vi "File-Generator Module.vi"(11 "Metadata for all trials/volumes":T1[](array[typedef])=[{"Imaging Protocol"=enum."Functional Acquisition", "Number of Trials"=2, "Frame Size"=512, "# Averaged frames"=1, "Dwell time (us)"=0.1, "Index of Z-plane"=0, "Timelapse?"=FALSE, "Logging process is active"=TRUE, "Speed logging enabled"=FALSE, "tdms file ref"=refnum, "path"=path "E:/UCL/Rig 3 MovCor integration version/Datasets/Dual Plane datasets/150701_01_13_28/Functional imaging TDMS data files/001.tdms", "Trial Number"=1, "Expected # points acquired"=TRUE, "Manually stopped"=FALSE, "Last trial"=FALSE, "Ch0 data"=[], "Ch1 data"=[], "Ref Data"=[], "Ref Frame Time"=[], "Image Time"=[], "Continuous Time"=[], "Ref X Length"=0, "Ref Y Length"=0, "# Ref Averaged frames"=1, "Ref Dwell time (us)"=0.20000000298023224, "Points acquired"={"Ch0 last trial"=34078720, "Ch1 last trial"=34078720, "All trials"=34078720}, "HW Timings File"=refnum}, {"Imaging Protocol"=enum."Functional Acquisition", "Number of Trials"=2, "Frame Size"=512, "# Averaged frames"=1, "Dwell time (us)"=0.1, "Index of Z-plane"=0, "Timelapse?"=FALSE, "Logging process is active"=TRUE, "Speed logging enabled"=FALSE, "tdms file ref"=refnum, "path"=path "E:/UCL/Rig 3 MovCor integration version/Datasets/Dual Plane datasets/150701_01_13_28/Functional imaging TDMS data files/002.tdms", "Trial Number"=2, "Expected # points acquired"=TRUE, "Manually stopped"=FALSE, "Last trial"=TRUE, "Ch0 data"=[], "Ch1 data"=[], "Ref Data"=[], "Ref Frame Time"=[], "Image Time"=[], "Continuous Time"=[], "Ref X Length"=0, "Ref Y Length"=0, "# Ref Averaged frames"=1, "Ref Dwell time (us)"=0.20000000298023224, "Points acquired"={"Ch0 last trial"=34078720, "Ch1 last trial"=34078720, "All trials"=68157440}, "HW Timings File"=refnum}, {"Imaging Protocol"=enum."Functional Acquisition", "Number of Trials"=2, "Frame Size"=512, "# Averaged frames"=1, "Dwell time (us)"=0.1, "Index of Z-plane"=0, "Timelapse?"=FALSE, "Logging process is active"=TRUE, "Speed logging enabled"=FALSE, "tdms file ref"=refnum, "path"=path "E:/UCL/Rig 3 MovCor integration version/Datasets/Dual Plane datasets/150701_01_13_28/Functional imaging TDMS data files/003.tdms", "Trial Number"=2, "Expected # points acquired"=TRUE, "Manually stopped"=FALSE, "Last trial"=TRUE, "Ch0 data"=[], "Ch1 data"=[], "Ref Data"=[], "Ref Frame Time"=[], "Image Time"=[], "Continuous Time"=[], "Ref X Length"=0, "Ref Y Length"=0, "# Ref Averaged frames"=1, "Ref Dwell time (us)"=0.20000000298023224, "Points acquired"={"Ch0 last trial"=34078720, "Ch1 last trial"=34078720, "All trials"=68157440}, "HW Timings File"=refnum}] {"Ref Dwell time (us)" format="%#.6g"; "Frame Size" items=["100X100"=100, "128X128"=128, "200X200"=200, "256X256"=256, "512X512"=512, "1024x1024"=1024, "2048x2048"=2048]; "Dwell time (us)" format="%#.6g"}) -> ()   [LabVIEW 2020]
uses:
  Typedefs/Logging queue element.ctl
  Typedefs/Imaging Protocols enum.ctl
  Typedefs/Frame Size.ctl
  Typedefs/Acquired points count.ctl
  Typedefs/Top level VI states.ctl
  Global Variables/General Globals.vi
  Global Variables/gl_Queues.vi
panel:
  out "Continuous Time":u64[][](array[numeric])
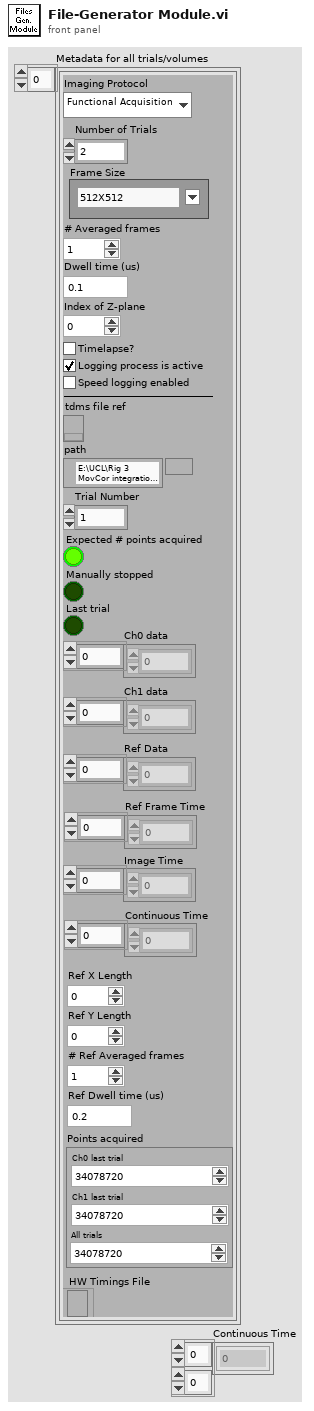
[diagram p1: front panel]
types:
  T1 = typedef "Logging queue element.ctl" = cluster{"Imaging Protocol":T2, "Number of Trials":u16, "Frame Size":T3, "# Averaged frames":u16, "Dwell time (us)":dbl, "Index of Z-plane":i32, "Timelapse?":bool, "Logging process is active":bool, "Speed logging enabled":bool, "tdms file ref":refnum<k34>, "path":path, "Trial Number":i32, "Expected # points acquired":bool, "Manually stopped":bool, "Last trial":bool, "Ch0 data":u32[], "Ch1 data":u32[], "Ref Data":u32[], "Ref Frame Time":u64[], "Image Time":u64[], "Continuous Time":u64[], "Ref X Length":u16, "Ref Y Length":u16, "# Ref Averaged frames":u16, "Ref Dwell time (us)":dbl, "Points acquired":T4, "HW Timings File":refnum<file>}
  T2 = typedef "Imaging Protocols enum.ctl" = enum16{"AOL Z-Stack", "Motor Z Stack", "Functional Acquisition", "Single Plane Acquisition", "Volume Acquisition", "Live Imaging", "Live Plane Imaging", "Live Volume Imaging"}
  T3 = typedef "Frame Size.ctl" = u16
  T4 = typedef "Acquired points count.ctl" = cluster{"Ch0 last trial":u64, "Ch1 last trial":u64, "All trials":u64}
  T5 = typedef "Top level VI states.ctl" = enum16{"None", "Initialise UI", "<STACK PROTOCOL STATES>", "AOL Zstack-START", "AOL Zstack-STOP", "Motor Zstack-START", "Motor Zstack-STOP", "<ACQUISITION PROTOCOL STATES> ", "Functional Acquisition-START", "Functional Acquisition-STOP", "Single Plane Acquisition-START", "Single Plane Acquisition-STOP", "Volume Acquisition-START", "Volume Acquisition-STOP", "<LIVE IMAGING PROTOCOL STATES>", "Live Imaging-START", "Live Imaging-STOP", "Live Plane Imaging-START", "Live Plane Imaging-STOP", "Live Volume Imaging-START", "Live Volume Imaging-STOP", "<MOVEMENT CORRECTION PROTOCOL STATES>", "EXIT"}
  T6 = typedef "All Message Queues.ctl" = cluster{"UI queue":refnum<queue>, "Acq. queue":refnum<queue>, "Logging queue":refnum<queue>}
  T7 = typedef "ROI ID Enum.ctl" = enum16{"Point", "MiniScan", "Comp. MiniScan", "Rectangle", "Comp. volume", "Arb. plane point", "None"}
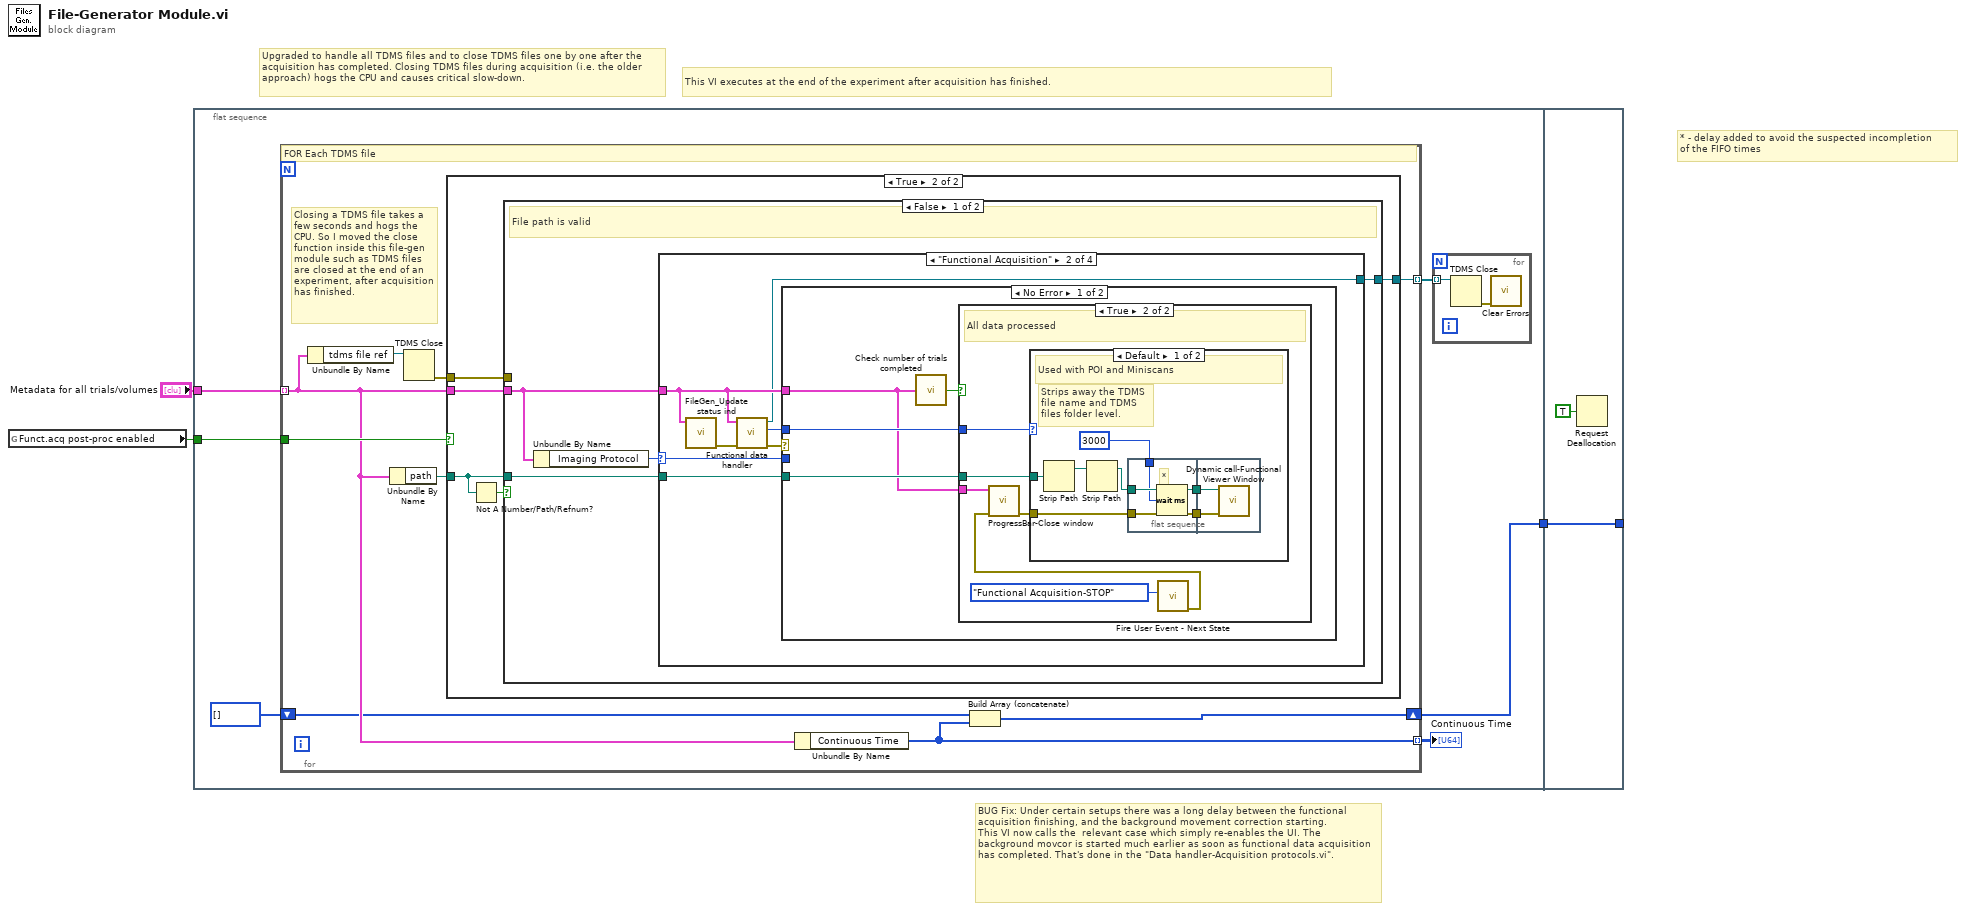
[diagram p0: block diagram]
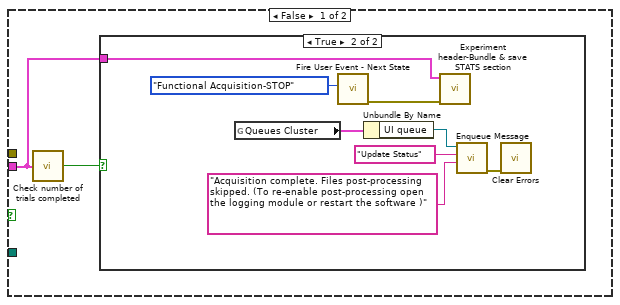
[diagram p2: hidden frame]
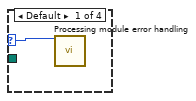
[diagram p4: hidden frame]
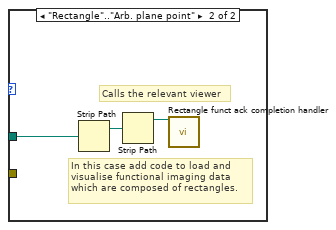
[diagram p6: hidden frame]
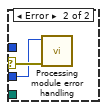
[diagram p7: hidden frame]
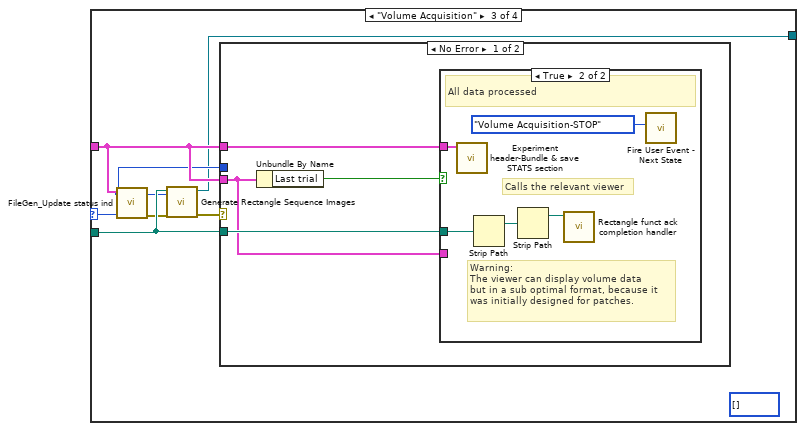
[diagram p8: hidden frame]
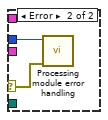
[diagram p10: hidden frame]
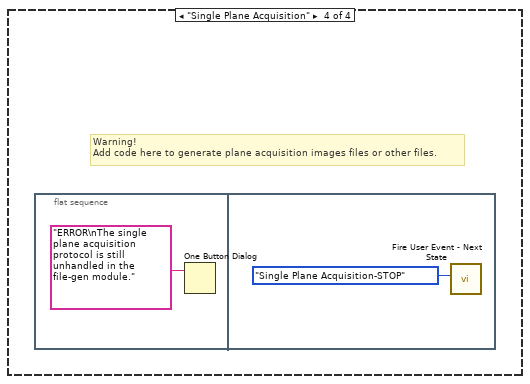
[diagram p11: hidden frame]
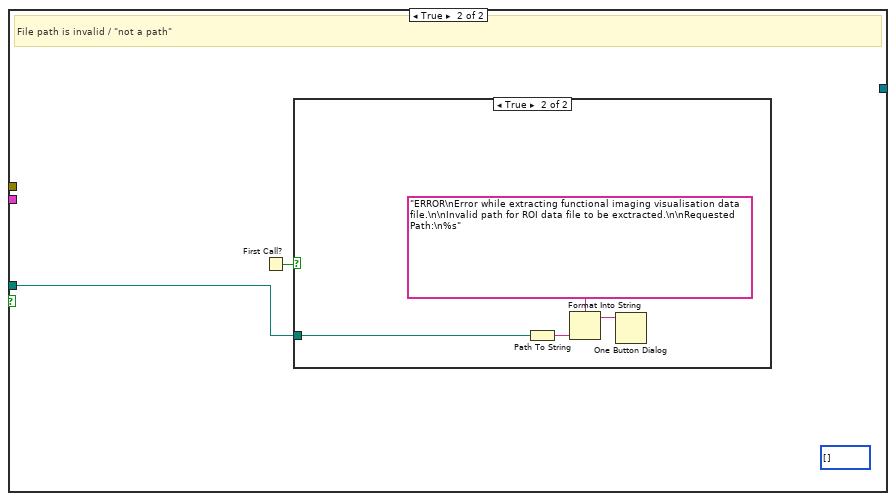
[diagram p12: hidden frame]
diagram:
  # "* - delay added to avoid the suspected incompletion\nof the FIFO times"
  # "BUG Fix: Under certain setups there was a long delay between the functional acquisition finishing, and the background movement correction starting.\nThis VI now calls the  relevant case which simply re-enables the UI. The background movcor is started much earlier as soon as functional data acquisition has completed. That's done in the \"Data handler-Acquisition protocols.vi\"."
  # "This VI executes at the end of the experiment after acquisition has finished."
  # "Upgraded to handle all TDMS files and to close TDMS files one by one after the acquisition has completed. Closing TDMS files during acquisition (i.e. the older approach) hogs the CPU and causes critical slow-down."
  n1 = global read "General Globals.vi" "Funct.acq post-proc enabled"() -> (w2:bool)
  n2 = flat-sequence {
    tunnel: "Metadata for all trials/volumes" -> [w9]
    tunnel: w2 -> [w8]
    tunnel: [w5] -> w1
    tunnel: [w100] -> _
    tunnel: w1 -> [w100]
    frame #0 {
      n3 = for {
        tunnel: w9 -> [w15] mode=indexing
        tunnel: w8 -> [w17]
        tunnel: [w16] -> w7 mode=indexing
        shift-right: [w13] -> w5
        shift-left: u64[] [] -> [w14]
        tunnel: [w12] -> w4 mode=indexing
        # "Closing a TDMS file takes a few seconds and hogs the CPU. So I moved the close function inside this file-gen module such as TDMS files are closed at the end of an experiment, after acquisition has finished."
        # "FOR Each TDMS file"
        n4 = Unbundle By Name(w15) -> ("tdms file ref"=w19:refnum<k34>)
        n5 = Unbundle By Name(w15) -> ("path"=w20:path)
        n6 = TDMS Close(11:w19) -> (0:w18:errorcluster)  [unwired: 1 in, 1 out]
        n7 = case shown="True" w17 {
          tunnel: w20 -> [_ w35]
          tunnel: w15 -> [w21 w34]
          tunnel: w18 -> [_ w33]
          tunnel: [_ w31] -> w16
          frame False {
            n8 = call "Check number of trials completed.vi"("Cluster"=w21) -> ("# of trials completed"=w22:bool)
            n9 = case shown="True" w22 {
              tunnel: w21 -> [_ w23]
              frame False {
              }
              frame True {
                n10 = global read "gl_Queues.vi" "Queues Cluster"() -> (w28:T6)
                n11 = call "Fire User Event - Next State.vi"("\"UI Handler loop\" case to execute"=Top_level_VI_states."Functional Acquisition-STOP" ("event data / imaging mode")) -> ("Error Out"=w24:errorcluster)  [unwired: 10 in]
                n12 = Unbundle By Name(w28) -> ("UI queue"=w27:refnum<queue>)
                n13 = call "Experiment header-Bundle & save STATS section.vi"("error in (no error)"=w24, "Logging queue element"=w23) -> ()  [unwired: 9 in, 1 out]
                n14 = call "Enqueue Message.vi"("Message Data"="Acquisition complete. Files post-processing skipped. (To re-enable post-processing open the logging module or restart the software )" ("Acquiring and Logging..."), "Message"="Update Status", "Queue"=w27) -> ("error out"=w26:errorcluster)  [unwired: 7 in, 1 out]
                n15 = call <vilib>:"Clear Errors.vi"("error in (no error)"=w26) -> ()  [unwired: 5 in, 2 out]
              }
            }
          }
          frame True {
            n16 = Not A Number/Path/Refnum?(number/path/refnum=w35) -> (NaN/Path/Refnum?=w32:bool)
            n17 = case shown="False" w32 {
              tunnel: w35 -> [w39 w95]
              tunnel: w34 -> [w37 _]
              tunnel: w33 -> [_ _]
              tunnel: [w36 _] -> w31
              frame False {
                # "File path is valid"
                n18 = Unbundle By Name(w37) -> ("Imaging Protocol"=w38:T2)
                n19 = case shown="\"Functional Acquisition\"" w38 {
                  selector: w38 -> [w40 w42 w76 _]
                  tunnel: w37 -> [_ w43 w77 _]
                  tunnel: w39 -> [_ w46 w80 _]
                  tunnel: [_ w41 w75 _] -> w36
                  frame Default {
                    n20 = call "Processing module error handling.vi"("Imaging Protocol"=w40) -> ()  [unwired: 11 in]
                  }
                  frame "Functional Acquisition" {
                    n21 = call "FileGen_Update status ind.vi"("Cluster"=w43) -> ("error out"=w44:errorcluster)  [unwired: 10 in]
                    n22 = call "Functional data handler.vi"("error in"=w44, "Setup cluster"=w43) -> ("error out"=w47:errorcluster, "Predominant ROI type"=w45:T7, "tdms file to close"=w41:refnum<k34>)  [unwired: 6 in, 1 out]
                    n23 = case shown="No Error" w47 {
                      selector: w47 -> [_ w74]
                      tunnel: w46 -> [w50 _]
                      tunnel: w43 -> [w48 _]
                      tunnel: w45 -> [w49 _]
                      tunnel: w42 -> [_ w73]
                      frame No Error {
                        n24 = call "Check number of trials completed.vi"("Cluster"=w48) -> ("# of trials completed"=w51:bool)
                        n25 = case shown="True" w51 {
                          tunnel: w50 -> [_ w57]
                          tunnel: w48 -> [_ w55]
                          tunnel: w49 -> [_ w56]
                          frame False {
                            # "Still processing..."
                          }
                          frame True {
                            # "All data processed"
                            n26 = call "Fire User Event - Next State.vi"("\"UI Handler loop\" case to execute"=Top_level_VI_states."Functional Acquisition-STOP" ("event data / imaging mode")) -> ("Error Out"=w52:errorcluster)  [unwired: 10 in]
                            n27 = call "ProgressBar-Close window.vi"("error in"=w52, "Z-stack queue cluster"=w55) -> ("error out (no error)"=w53:errorcluster)  [unwired: 9 in]
                            n28 = case shown="Default" w56 {
                              tunnel: w57 -> [w63 w71]
                              tunnel: w53 -> [w62 _]
                              frame Default {
                                # "Strips away the TDMS file name and TDMS files folder level."
                                # "Used with POI and Miniscans"
                                n29 = Strip Path(path=w63) -> (stripped path=w64:path)  [unwired: 1 out]
                                n30 = Strip Path(path=w64) -> (stripped path=w61:path)  [unwired: 1 out]
                                n31 = flat-sequence {
                                tunnel: w61 -> [w66]
                                tunnel: w62 -> [w67]
                                tunnel: [w67] -> w60
                                tunnel: [w66] -> w59
                                tunnel: u32 3000 -> [w65]
                                tunnel: w60 -> [w69]
                                tunnel: w59 -> [w68]
                                frame #0 {
                                # "*"
                                n32 = Wait (ms)(milliseconds to wait=w65) -> ()  [unwired: 1 out]
                                }
                                frame #1 {
                                n33 = call "Dynamic call-Functional Viewer Window.vi"("error in (no error)"=w69, "Experiment data folder path"=w68) -> ()  [unwired: 10 in]
                                }
                                }
                              }
                              frame "Rectangle".."Arb. plane point" {
                                # "Calls the relevant viewer"
                                # "In this case add code to load and visualise functional imaging data which are composed of rectangles."
                                n34 = Strip Path(path=w71) -> (stripped path=w72:path)  [unwired: 1 out]
                                n35 = Strip Path(path=w72) -> (stripped path=w70:path)  [unwired: 1 out]
                                n36 = call "Rectangle funct ack completion handler.vi"("Destination folder"=w70) -> ()  [unwired: 11 in]
                              }
                            }
                          }
                        }
                      }
                      frame Error {
                        n37 = call "Processing module error handling.vi"("error in (no error)"=w74, "Imaging Protocol"=w73) -> ()  [unwired: 10 in]
                      }
                    }
                  }
                  frame "Volume Acquisition" {
                    (unwired) u64[] [] ("Continuous Time")
                    n38 = call "FileGen_Update status ind.vi"("Cluster"=w77) -> ("error out"=w78:errorcluster)  [unwired: 10 in]
                    n39 = call "Generate Rectangle Sequence Images.vi"("Imaging Protocol"=w76, "error in (no error)"=w78, "TDMS file path & name"=w80) -> ("error out"=w79:errorcluster, "tdms file to close"=w75:refnum<k34>)  [unwired: 6 in, 1 out]
                    n40 = case shown="No Error" w79 {
                      selector: w79 -> [_ w91]
                      tunnel: w80 -> [w84 _]
                      tunnel: w77 -> [w83 _]
                      tunnel: w77 -> [w81 _]
                      tunnel: w76 -> [_ w90]
                      frame No Error {
                        n41 = Unbundle By Name(w83) -> ("Last trial"=w82:bool)
                        n42 = case shown="True" w82 {
                          tunnel: w84 -> [_ w85]
                          tunnel: w83 -> [_ _]
                          tunnel: w81 -> [_ w88]
                          frame False {
                            # "Still processing..."
                          }
                          frame True {
                            # "Warning:\nThe viewer can display volume data\nbut in a sub optimal format, because it\nwas initially designed for patches."
                            # "Calls the relevant viewer"
                            # "All data processed"
                            n43 = call "Experiment header-Bundle & save STATS section.vi"("Logging queue element"=w88) -> ()  [unwired: 10 in, 1 out]
                            n44 = Strip Path(path=w85) -> (stripped path=w87:path)  [unwired: 1 out]
                            n45 = Strip Path(path=w87) -> (stripped path=w86:path)  [unwired: 1 out]
                            n46 = call "Rectangle funct ack completion handler.vi"("Destination folder"=w86) -> ()  [unwired: 11 in]
                            n47 = call "Fire User Event - Next State.vi"("\"UI Handler loop\" case to execute"=Top_level_VI_states."Volume Acquisition-STOP" ("event data / imaging mode")) -> ()  [unwired: 10 in, 1 out]
                          }
                        }
                      }
                      frame Error {
                        n48 = call "Processing module error handling.vi"("error in (no error)"=w91, "Imaging Protocol"=w90) -> ()  [unwired: 10 in]
                      }
                    }
                  }
                  frame "Single Plane Acquisition" {
                    # "Warning!\nAdd code here to generate plane acquisition images files or other files."
                    n49 = flat-sequence {
                      frame #0 {
                        n50 = One Button Dialog(message="ERROR\nThe single plane acquisition protocol is still unhandled in the file-gen module.") -> ()  [unwired: 1 in, 1 out]
                      }
                      frame #1 {
                        n51 = call "Fire User Event - Next State.vi"("\"UI Handler loop\" case to execute"=Top_level_VI_states."Single Plane Acquisition-STOP" ("event data / imaging mode")) -> ()  [unwired: 10 in, 1 out]
                      }
                    }
                  }
                }
              }
              frame True {
                (unwired) u64[] [] ("Continuous Time")
                # "File path is invalid / \"not a path\""
                n52 = First Call?() -> (First Call?: T/F=w94:bool)
                n53 = case shown="True" w94 {
                  tunnel: w95 -> [_ w99]
                  frame False {
                  }
                  frame True {
                    n54 = Path To String(path=w99) -> (string=w97:string)
                    n55 = Format Into String(format string="ERROR\nError while extracting functional imaging visualisation data file.\n\nInvalid path for ROI data file to be exctracted.\n\nRequested Path:\n%s", w97) -> (resulting string=w96:string)  [unwired: 2 in, 1 out]
                    n56 = One Button Dialog(message=w96) -> ()  [unwired: 1 in, 1 out]
                  }
                }
              }
            }
          }
        }
        n57 = Unbundle By Name(w15) -> ("Continuous Time"=w12:u64[])
        n58 = Build Array (concatenate)(w14, w12) -> (w13:u64[])
      }
      "Continuous Time" <- w4
      n59 = for {
        tunnel: w7 -> [w11] mode=indexing
        n60 = TDMS Close(11:w11) -> (0:w10:errorcluster)  [unwired: 1 in, 1 out]
        n61 = call <vilib>:"Clear Errors.vi"("error in (no error)"=w10) -> ()  [unwired: 5 in, 2 out]
      }
    }
    frame #1 {
      n62 = Request Deallocation(TRUE ("flag")) -> ()
    }
  }
